vi "Host.vi"() -> ()   [LabVIEW 2025]
uses:
  <vilib>/Analysis/baseanly.llb/Real Dot Product.vi
  <vilib>/Analysis/baseanly.llb/Real A x B.vi
  <vilib>/Analysis/Matrix/Numeric/Conversions/Matrix To Array - RM.vi
  <vilib>/FPGAPlugInAG/cRIO-9033/niLvFpga_Open_cRIO-9033.vi
  <vilib>/rvi/interface/common/dynamic/niFpgaDynamicAddResources.vi
  <vilib>/Utility/error.llb/Error Cluster From Error Code.vi
  <vilib>/rvi/errors/niLvFpgaAdjustHostInterfaceError.vi
  <vilib>/FPGAPlugInAG/Dynamic/niLvFpga_Run_Dynamic.vi
  <vilib>/FPGAPlugInAG/Dynamic/niLvFpga_Close_Dynamic.vi
  <vilib>/rvi/interface/nirviOpenFPGA/nirviOpenFPGA.xnode
  FPGA Bitfiles/dotplot9033_FPGATarget_Target_CwM8WDNFVFM.lvbitx
  Target.vi
  <vilib>/rvi/interface/nirviMethod/nirviMethod.xnode
  <vilib>/rvi/interface/nirviCloseFPGA/nirviCloseFPGA.xnode
  <vilib>/FPGAPlugInAG/Dynamic/niLvFpga_WriteFifo_Dynamic.vi
  <vilib>/rvi/errors/niLvFpgaMergeErrorWithErrorCode.vi
  <vilib>/Analysis/NI_AALBase.lvlib
  <vilib>/Analysis/Matrix/NI_Matrix.lvlib
  <vilib>/FPGAPlugInAG/Dynamic/niLvFpga_ReadFifo_Dynamic.vi
panel:
  out "X * Y":dbl format="%.6f"
  out "elements in B":i32
  out "elements in A":i32
  out "sum of error":dbl
  out "C - FPGA code":sgl[][](array[numeric])
  out "elements in C":i32
  out "C - Real":dbl[][](array[numeric])
  out "B":sgl[][](array[numeric])
  out "A":sgl[][](array[numeric])
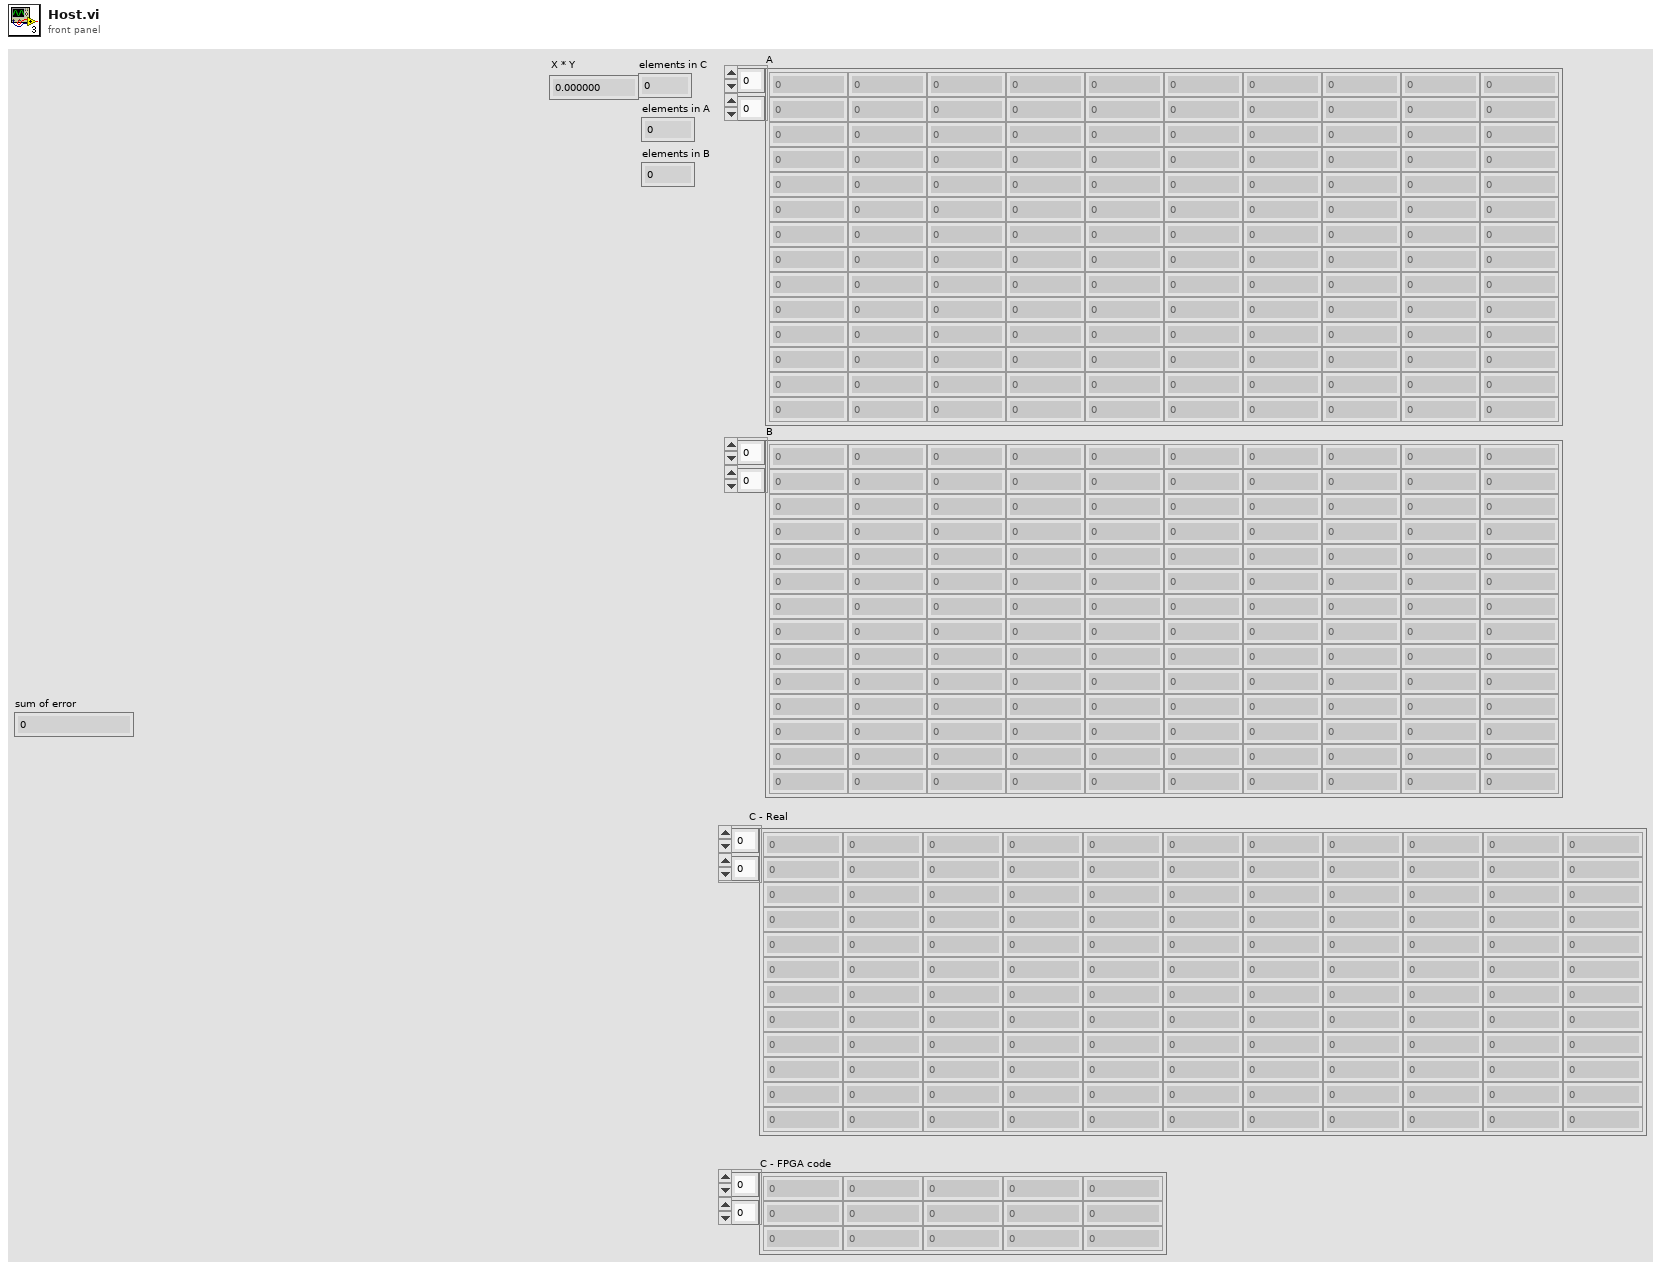
[diagram p1: front panel]
types:
  T1 = typedef "NI_Matrix.lvlib/RealMatrix.ctl" = dbl[][]
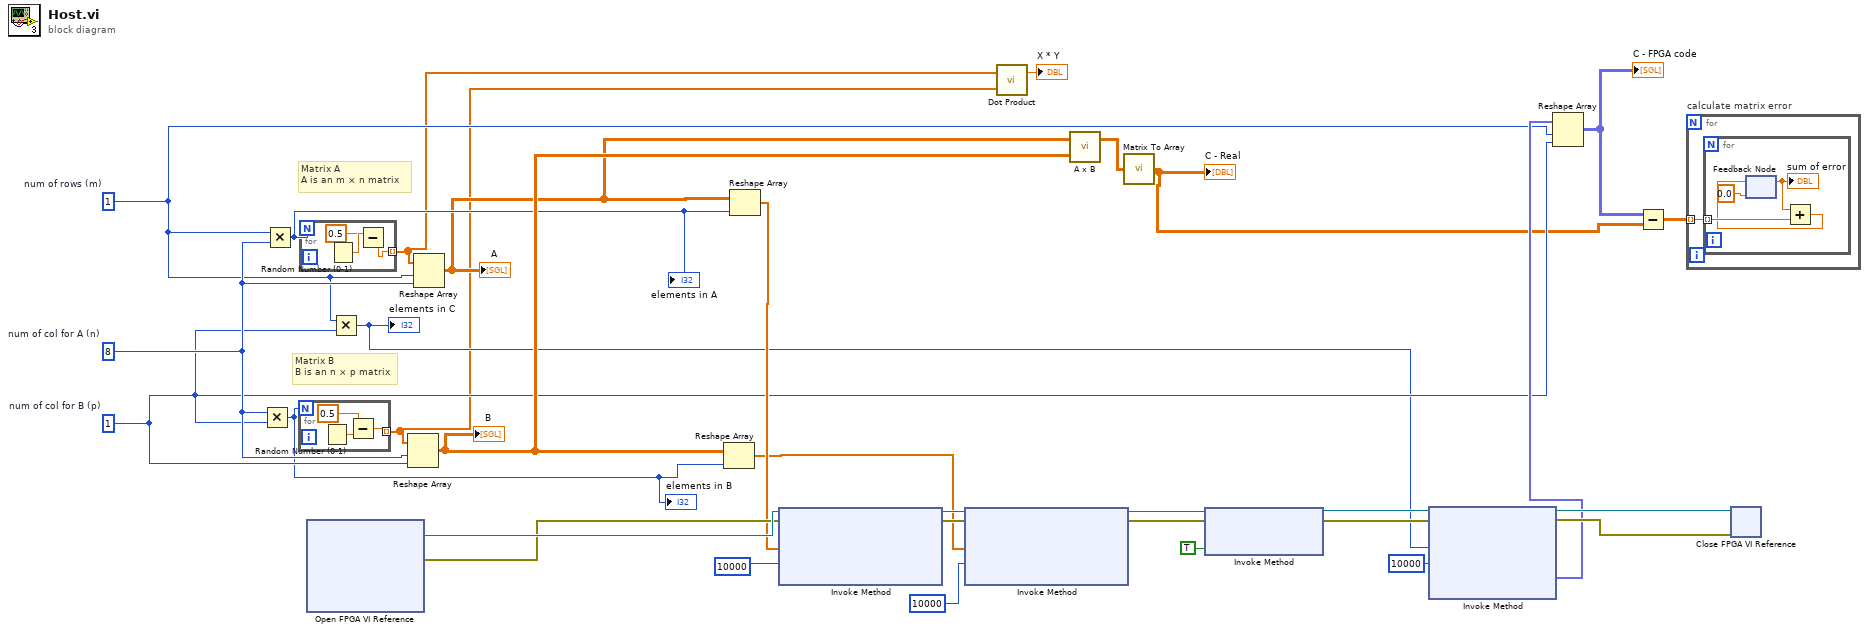
[diagram p0: block diagram]
diagram:
  w11 = 1  # num of col for B (p)
  w18 = 8  # num of col for A (n)
  w12 = 1  # num of rows (m)
  # "Matrix B\nB is an n × p matrix"
  # "Matrix A\nA is an m × n matrix"
  n1 = Multiply(x=w18, y=w11) -> (x*y=w8:i32)
  "elements in B" <- w8
  n2 = Multiply(x=w12, y=w18) -> (x*y=w19:i32)
  "elements in A" <- w19
  n3 = for {
    N: w8 -> [_]
    tunnel: [w34] -> w5 mode=indexing
    n4 = Random Number (0-1)() -> (number: 0 to 1=w35:dbl)
    n5 = Subtract(x=w35, y=sgl 0.5) -> (x-y=w34:sgl)
  }
  n6 = for {
    N: w19 -> [_]
    tunnel: [w37] -> w6 mode=indexing
    n7 = Random Number (0-1)() -> (number: 0 to 1=w38:dbl)
    n8 = Subtract(x=w38, y=sgl 0.5) -> (x-y=w37:sgl)
  }
  n9 = xnode "Open FPGA VI Reference"() -> ("FPGA VI Reference Out"=w31:refnum<k20>, "error out"=w30:errorcluster)  [unwired: 2 in]
  n10 = Multiply(x=w12, y=w11) -> (x*y=w9:i32)
  "elements in C" <- w9
  n11 = Reshape Array(w5, w18, w11) -> (w21:sgl[][])
  "B" <- w21
  n12 = Reshape Array(w6, w12, w18) -> (w7:sgl[][])
  "A" <- w7
  n13 = Reshape Array(w21, w8) -> (w16:sgl[])
  n14 = Reshape Array(w7, w19) -> (w17:sgl[])
  n15 = xnode "Invoke Method"("FPGA VI Reference In"=w31, "error in"=w30, "Data"=w17, "Timeout (ms)"=10000) -> ("FPGA VI Reference Out"=w25:refnum<k20>, "error out"=w24:errorcluster)  [unwired: 1 out]
  n16 = xnode "Invoke Method"("FPGA VI Reference In"=w25, "error in"=w24, "Data"=w16, "Timeout (ms)"=10000) -> ("FPGA VI Reference Out"=w23:refnum<k20>, "error out"=w22:errorcluster)  [unwired: 1 out]
  n17 = call-poly <vilib>:"Dot Product.vi"("Y Vector"=w5, "X Vector"=w6) -> ("X * Y"=→"X * Y":dbl)  [unwired: 1 out]
  n18 = call-poly <vilib>:"A x B.vi"("B"=w21, "A"=w7) -> ("A x B"=w20:T1)  [unwired: 1 out]
  n19 = call-poly <vilib>:"Matrix To Array.vi"("Real Matrix"=w20) -> ("Real 2D Array"=w10:dbl[][])
  "C - Real" <- w10
  n20 = xnode "Invoke Method"("FPGA VI Reference In"=w23, "error in"=w22, "Wait Until Done (F)"=TRUE) -> ("FPGA VI Reference Out"=w29:refnum<k20>, "error out"=w28:errorcluster)
  n21 = xnode "Invoke Method"("FPGA VI Reference In"=w29, "error in"=w28, "Number of Elements"=w9, "Timeout (ms)"=10000) -> ("FPGA VI Reference Out"=w27:refnum<k20>, "error out"=w26:errorcluster, "Data"=w13:fxp<+/-,32,16>[])  [unwired: 1 out]
  n22 = Reshape Array(w13, w12, w11) -> (w15:fxp<+/-,32,16>[][])
  "C - FPGA code" <- w15
  n23 = Subtract(x=w15, y=w10) -> (x-y=w14:dbl[][])
  n24 = for "calculate matrix error" {
    tunnel: w14 -> [w39] mode=indexing
    n25 = for {
      tunnel: w39 -> [w43] mode=indexing
      n26 = feedback #1(0.0) -> (w41:dbl)
      "sum of error" <- w41
      n27 = Add(x=w41, y=w43) -> (x+y=w42:dbl)
      n28 = feedback-in #1(w42) -> ()
    }
  }
  n29 = xnode "Close FPGA VI Reference"("FPGA VI Reference In"=w27, "error in"=w26) -> ()  [unwired: 1 out]
